vi "DmgrClose.vi"(8 "Error In":errorcluster, 11 "hif":u32) -> (0 "Error Out":errorcluster)   [LabVIEW 2011, in "LVH-Adept.lvlib" / "DMGR.lvlib"]
uses:
  DMGR.lvlib
  Resources/dmgr.dll
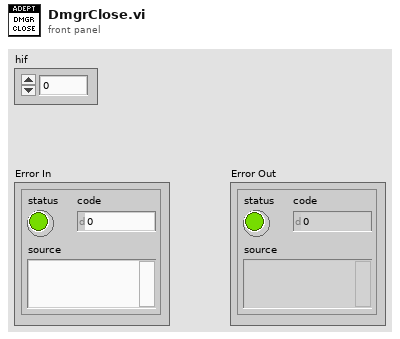
[diagram p1: front panel]
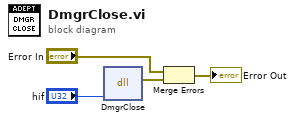
[diagram p0: block diagram]
diagram:
  n1 = dll-call lib="C:/github/makerhub/Adept/LabVIEW/vi.lib/MakerHub/Adept/Private/Resources/dmgr.dll" fn="DmgrClose"("hif"="hif") -> (error out=w1:errorcluster)  [unwired: 5 in, 1 out]
  n2 = Merge Errors("Error In", w1) -> (→"Error Out":errorcluster)
